vi "pointers.vi"() -> ()   [LabVIEW 2013]
uses:
  cvibuild.LabVIEW MQTT/Debug/LabVIEW MQTT.dll
panel:
  out "v 2":i32
  out "p 2":i32
  out "h 2":i32
  out "return type 2":i32
  out "error out":errorcluster
  in  "v":i32
  in  "p":i32
  in  "h":i32
  in  "return type":i32
  in  "error in (no error)":errorcluster
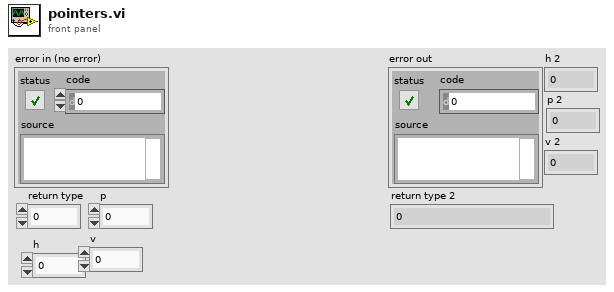
[diagram p1: front panel]
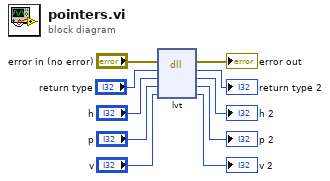
[diagram p0: block diagram]
diagram:
  n1 = dll-call lib="C:/Users/Daniel/Desktop/MQTT CVI/cvibuild.LabVIEW MQTT/Debug/LabVIEW MQTT.dll" fn="lvt"(error in="error in (no error)", "return type"="return type", "h"="h", "p"="p", "v"="v") -> (error out=→"error out":errorcluster, "return type"=→"return type 2":i32, "h"=→"h 2":i32, "p"=→"p 2":i32, "v"=→"v 2":i32)  [unwired: 1 in, 1 out]
